vi "Execution_MessageHandler_AddMessageToLog.vi"(8 "error in (no error)":errorcluster, 10 "Messages.lvclass":refnum<class "Messages.lvclass">, 11 "MessageHandler.lvclass in":refnum<class "MessageHandler.lvclass">) -> (0 "error out":errorcluster, 3 "MessageHandler.lvclass out":refnum<class "MessageHandler.lvclass">)   [LabVIEW 2013, in "MessageHandler.lvclass"]
uses:
  Class/MessageHandler.lvclass
  050 - CONFIG/00 - ApplicationConfig/Ctrls/EnumFgvConfigCommand.ctl
  001 - MAIN/Class/Messages/ErrorMessage/ErrorMessage.lvclass
  001 - MAIN/Class/Messages/Messages.lvclass
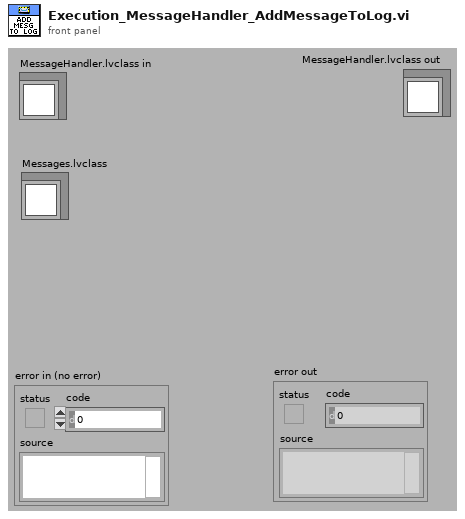
[diagram p1: front panel]
types:
  T1 = typedef "EnumFgvConfigCommand.ctl" = enum16{"Load", "Get", "Set", "Save To Disk"}
  T2 = typedef "ApplicationConfig.ctl" = cluster{"Data Path":path, "MessageHandlerConfig":T3, "Simulation":bool, "Dictionnary":string}
  T3 = typedef "MessageHandlerConfig.ctl" = cluster{"Max log files":u32, "Max messages per file":u32}
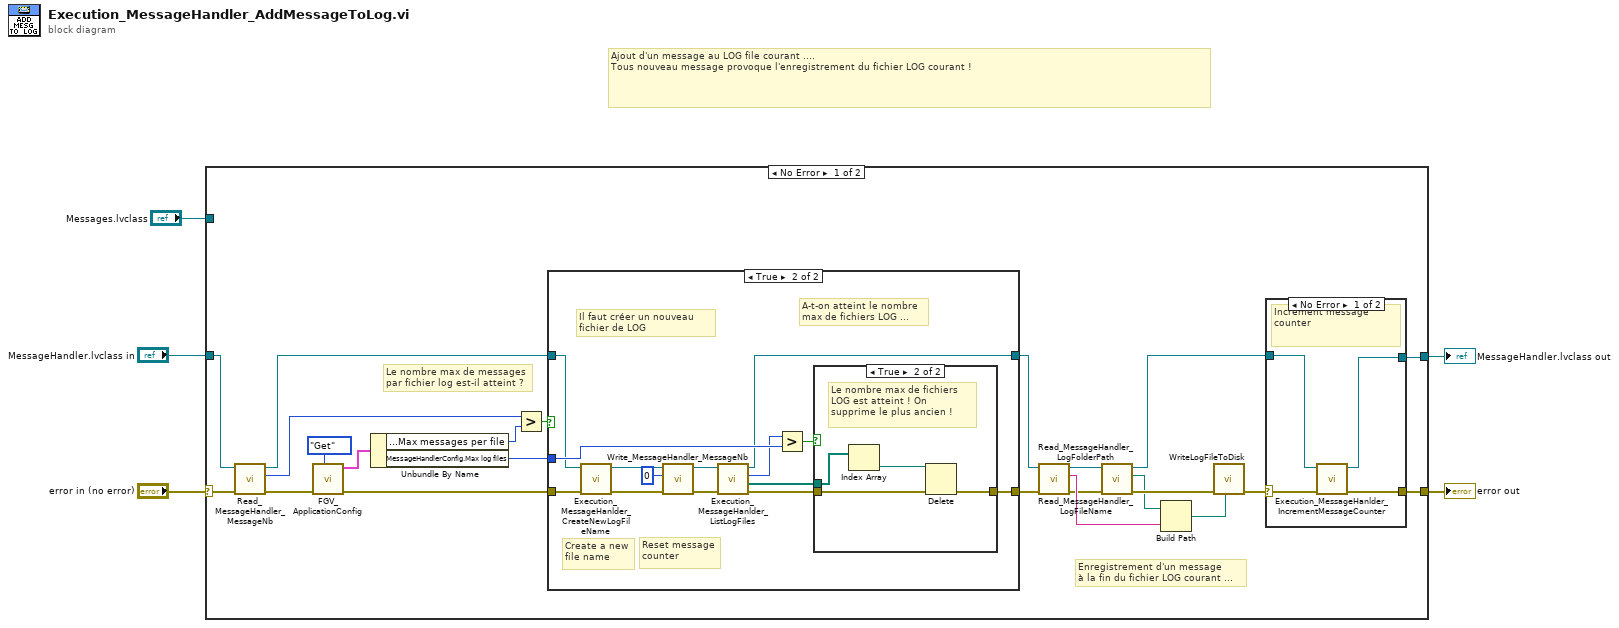
[diagram p0: block diagram]
diagram:
  # "Ajout d'un message au LOG file courant ....\nTous nouveau message provoque l'enregistrement du fichier LOG courant !"
  n1 = case shown="No Error" "error in (no error)" {
    selector: "error in (no error)" -> [w18 w57]
    tunnel: [w20 w57] -> w4
    tunnel: "MessageHandler.lvclass in" -> [w14 w56]
    tunnel: [w19 w56] -> w2
    tunnel: "Messages.lvclass" -> [_ _]
    frame No Error {
      # "Enregistrement d'un message\nà la fin du fichier LOG courant ..."
      # "Le nombre max de messages\npar fichier log est-il atteint ?"
      n2 = call-dynamic "Read_MessageHandler_MessageNb.vi"("error in (no error)"=w18, "MessageHandler in"=w14) -> ("error out"=w17:errorcluster, "Message number"=w16:u32, "MessageHandler out"=w15:refnum<class "MessageHandler.lvclass">)  [unwired: 7 in]
      n3 = call "FGV_ApplicationConfig.vi"("Command"=EnumFgvConfigCommand."Get", "error in (no error)"=w17) -> ("error out"=w25:errorcluster, "ApplicationConfigOut"=w27:T2)  [unwired: 8 in]
      n4 = Unbundle By Name(w27) -> ("MessageHandlerConfig.Max messages per file"=w26:u32, "MessageHandlerConfig.Max log files"=w22:u32)
      n5 = Greater?(x=w16, y=w26) -> (0:w24:bool)
      n6 = case shown="True" w24 {
        tunnel: w25 -> [w35 w47]
        tunnel: w15 -> [w36 w46]
        tunnel: [w36 w39] -> w12
        tunnel: [w35 w48] -> w13
        tunnel: w22 -> [_ w50]
        frame False {
          # "Le nombre max de messages\npar fichier n'est pas encore\natteint !"
        }
        frame True {
          # "Reset message\ncounter"
          # "Create a new\nfile name"
          # "A-t-on atteint le nombre\nmax de fichiers LOG ..."
          # "Il faut créer un nouveau\nfichier de LOG"
          n7 = call-dynamic "Execution_MessageHanlder_CreateNewLogFileName.vi"("error in (no error)"=w47, "MessageHandler in"=w46) -> ("error out"=w45:errorcluster, "MessageHandler out"=w44:refnum<class "MessageHandler.lvclass">)  [unwired: 8 in]
          n8 = call-dynamic "Write_MessageHandler_MessageNb.vi"("error in (no error)"=w45, "Message number"=u32 0, "MessageHandler in"=w44) -> ("error out"=w42:errorcluster, "MessageHandler out"=w40:refnum<class "MessageHandler.lvclass">)  [unwired: 7 in]
          n9 = call-dynamic "Execution_MessageHanlder_ListLogFiles.vi"("error in (no error)"=w42, "MessageHandler in"=w40) -> ("error out"=w41:errorcluster, "Log file paths"=w37:path[], "Log file nb"=w38:u32, "MessageHandler out"=w39:refnum<class "MessageHandler.lvclass">)  [unwired: 6 in]
          n10 = Greater?(x=w38, y=w50) -> (0:w49:bool)
          n11 = case shown="True" w49 {
            tunnel: w41 -> [w51 w54]
            tunnel: w37 -> [_ w55]
            tunnel: [w51 w53] -> w48
            frame False {
              # "Le nombre max de fichiers\nn'est pas atteint !"
            }
            frame True {
              # "Le nombre max de fichiers\nLOG est atteint ! On \nsupprime le plus ancien !"
              n12 = Index Array(array=w55) -> (element=w52:path)  [unwired: 1 in]
              n13 = Delete(path (use dialog)=w52, error in=w54) -> (error out=w53:errorcluster)  [unwired: 3 in, 2 out]
            }
          }
        }
      }
      n14 = call-dynamic "Read_MessageHandler_LogFileName.vi"("error in (no error)"=w13, "MessageHandler in"=w12) -> ("error out"=w10:errorcluster, "LogFileName"=w11:string, "MessageHandler out"=w7:refnum<class "MessageHandler.lvclass">)  [unwired: 7 in]
      n15 = call-dynamic "Read_MessageHandler_LogFolderPath.vi"("error in (no error)"=w10, "MessageHandler in"=w7) -> ("error out"=w9:errorcluster, "Log Folder Path"=w8:path, "MessageHandler out"=w6:refnum<class "MessageHandler.lvclass">)  [unwired: 7 in]
      n16 = Build Path(base path=w8, name or relative path=w11) -> (appended path=w23:path)
      n17 = call "WriteLogFileToDisk.vi"("Log File path"=w23, "error in (no error)"=w9) -> ("error out"=w21:errorcluster)  [unwired: 9 in]
      n18 = case shown="No Error" w21 {
        selector: w21 -> [w30 w33]
        tunnel: w6 -> [w32 w34]
        tunnel: [w29 w33] -> w20
        tunnel: [w31 w34] -> w19
        frame No Error {
          # "Increment message counter"
          n19 = call-dynamic "Execution_MessageHanlder_IncrementMessageCounter.vi"("error in (no error)"=w30, "MessageHandler in"=w32) -> ("error out"=w29:errorcluster, "MessageHandler out"=w31:refnum<class "MessageHandler.lvclass">)  [unwired: 8 in]
        }
        frame Error {
        }
      }
    }
    frame Error {
    }
  }
  "error out" <- w4
  "MessageHandler.lvclass out" <- w2
